vi "Generate call result event.vi"(8 "error in (no error)":errorcluster, 10 "ICallResult":refnum<class "ICallResult.lvclass">, 11 "JsonEvents in":refnum<class "JsonEvents.lvclass">) -> (0 "error out":errorcluster, 3 "JsonEvents out":refnum<class "JsonEvents.lvclass">)   [LabVIEW 2020, in "wamplv.lvlib" / "JsonEvents.lvclass"]
uses:
  JsonEvents.lvclass
  JsonEvents.lvclass/JsonEvents.ctl
  Requests/Call/CallResult JSON/CallResult JSON.lvclass
  Requests/Call/ICallResult/ICallResult.lvclass
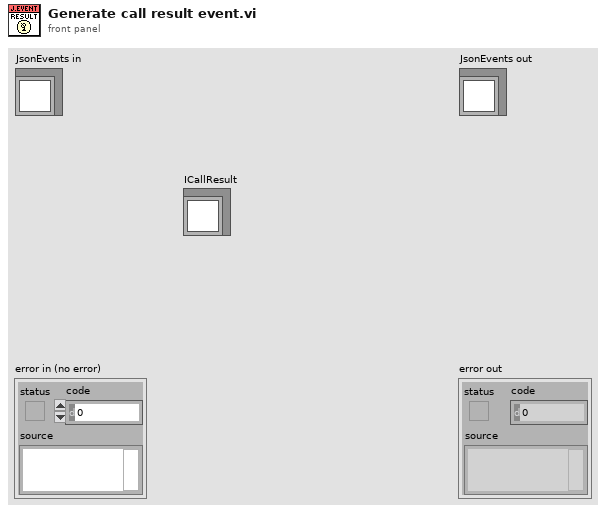
[diagram p1: front panel]
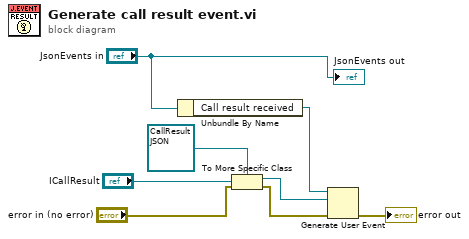
[diagram p0: block diagram]
diagram:
  n1 = Unbundle By Name("JsonEvents in") -> ("Call result received"=w3:refnum<user-event>)
  n2 = To More Specific Class(target class=refnum<class "CallResult JSON.lvclass"> refnum ("wamplv.lvlib:CallResult JSON.lvclass"), reference="ICallResult", error in="error in (no error)") -> (specific class reference=w4:refnum<class "CallResult JSON.lvclass">, error out=w6:errorcluster)
  n3 = Generate User Event(user event=w3, event data cluster=w4, error in=w6) -> (error out=→"error out":errorcluster)  [unwired: 1 in, 1 out]
  "JsonEvents out" <- "JsonEvents in"
